vi "cell simulator - REAL TIME.vi"() -> ()   [LabVIEW 2017]
panel:
  in  "Tab Control":enum32{"SIMULATION"}(tab)
  in  "OK Button":bool
  in  "simulation setup":T1={"Setup test by"=2, "config value"=4.0, "time unit of panel"=0} {"time unit of panel" items=["seconds(s)", "minutes(min)", "hours(h)"]; "Setup test by" items=["Time(s)", "Current(A)", "C discharge"]}
  out "simulation conditions":T2
  out "time test":i32 format="%<%H:%M:%S>t"
  in  "Cell characteristics":T3={"temperature(ªC)\nbattery not used "=0.0, "N cycles"=0.0, "Time cell\nnot used(months)"=0.0, "Cycling temperature\nto K factors"=0, "capacity cell(Ah)"=10.0} {"Cycling temperature\nto K factors" items=["25ºC", "50ºC"]}
  out "Losses of capacity":T4
  in  "?":enum32{"PRINCIPAL GRAPH", "GRAPH DETAILS"}(tab)
  out "SOC(%)":dbl(slide) scale=0.0..100.0
  out "resolucion  \nSOC % / 1s":dbl
  out "principal graph":dynamicdata(graph)
  out "Vbat graph":dbl(graph)
  out "SOC graph":dbl(graph)
  out "C graph":dbl(graph)
  out "Current graph":dbl(graph)
  # "Vbat(V)"
  # "SOC(/)"
  # "C rate"
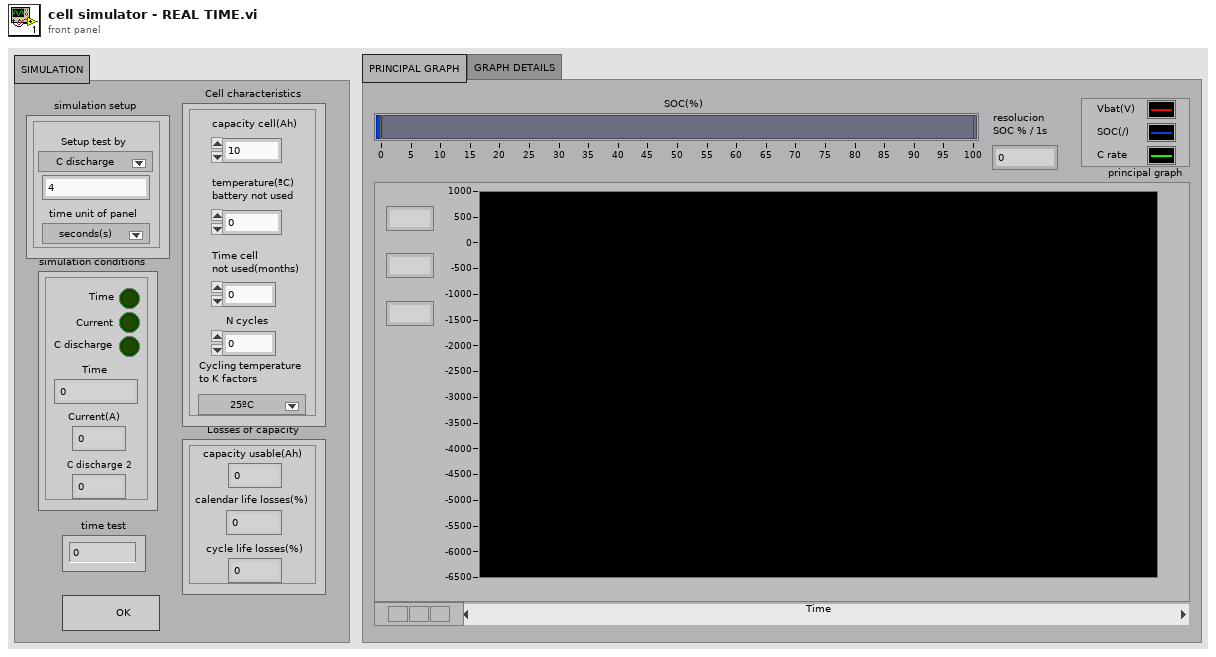
[diagram p1: front panel]
types:
  T1 = cluster{"Setup test by":u16, "config value":dbl, "time unit of panel":u16}
  T2 = cluster{"Time":bool, "Current":bool, "C discharge":bool, "Time":dbl, "Current(A)":dbl, "C discharge 2":dbl}
  T3 = cluster{"temperature(ªC)\nbattery not used ":dbl, "N cycles":dbl, "Time cell\nnot used(months)":dbl, "Cycling temperature\nto K factors":u16, "capacity cell(Ah)":dbl}
  T4 = cluster{"capacity usable(Ah)":dbl, "cycle life losses(%)":dbl, "calendar life losses(%)":dbl}
  T5 = cluster{" capacity usable(Ah)":dbl, " calendar life losses(%)":dbl, "cycle life losses(%)":dbl}
  T6 = cluster{"Time":bool, " Current":bool, "C discharge":bool, "Time(s)":dbl, "Current(A)":dbl, "C discharge":dbl}
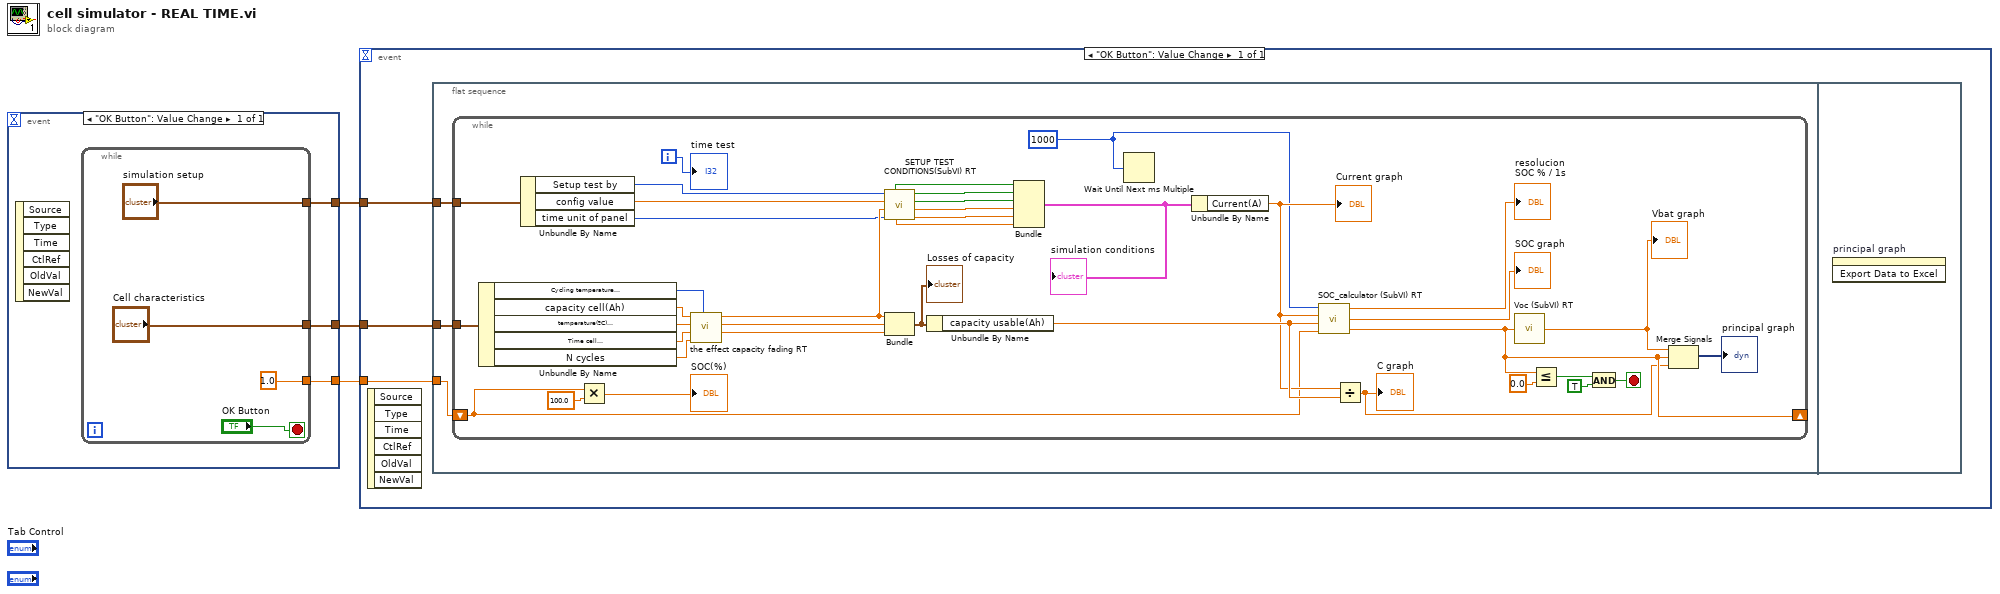
[diagram p0: block diagram]
diagram:
  n1 = event shown="[0] \"OK Button\": Value Change" {
    selector: _ -> [_]
    dyn-events: _ -> [_]
    timeout: _ -> [_]
    tunnel: [w6] -> w3
    tunnel: [w5] -> w2
    tunnel: [w4] -> w1
    event "OK Button": Value Change {
      n2 = event-data() -> ()  [unwired: 1 in, 6 out]
      n3 = while {
        tunnel: ["Cell characteristics"] -> w6
        tunnel: ["simulation setup"] -> w5
        tunnel: [1.0 ("Actual SOC( / )")] -> w4
        stop <- "OK Button" stop-if-true
      }
    }
  }
  n4 = event shown="[0] \"OK Button\": Value Change" {
    selector: _ -> [_]
    dyn-events: _ -> [_]
    timeout: _ -> [_]
    tunnel: w1 -> [w13]
    tunnel: w3 -> [w12]
    tunnel: w2 -> [w11]
    event "OK Button": Value Change {
      n5 = event-data() -> ()  [unwired: 1 in, 6 out]
      n6 = flat-sequence {
        tunnel: w13 -> [w16]
        tunnel: w12 -> [w15]
        tunnel: w11 -> [w14]
        frame #0 {
          n7 = while {
            shift-right: [w26] -> _
            shift-left: w16 -> [w24]
            tunnel: w15 -> [w30]
            tunnel: w14 -> [w29]
            i -> [w34]
            stop <- w27 stop-if-true
            w18 = u32 1000 ("millisecond multiple")
            n8 = Unbundle By Name(w30) -> ("Cycling temperature\nto K factors"=w52:u16, "capacity cell(Ah)"=w51:dbl, "temperature(ªC)\nbattery not used"=w50:dbl, "Time cell\nnot used(months)"=w49:dbl, "N cycles"=w48:dbl)
            n9 = Unbundle By Name(w29) -> ("Setup test by"=w47:u16, "config value"=w46:dbl, "time unit of panel"=w36:u16)
            n10 = Multiply(x=w24, y=100.0) -> (x*y=→"SOC(%)":dbl)
            n11 = call "the effect capacity fading RT.vi"("Cycling\ntemperature\nto K factors"=w52, "N cycles"=w48, "Time cell\nnot used(months)"=w49, "temperature(ªC) battery not used"=w50, "capacity cell"=w51) -> ("cycle life losses(%)"=w53:dbl, "calendar life losses(%)"=w54:dbl, "capacity usable(Ah)"=w45:dbl)  [unwired: 1 out]
            n12 = call "SETUP TEST CONDITIONS(SubVI) RT.vi"("setup time"=w36, "capacity usable(Ah)"=w45, "setup value"=w46, "setup test by"=w47) -> ("Current(A)"=w40:dbl, "Time(s)"=w41:dbl, 2:"C discharge"=w43:bool, "Current"=w44:bool, 4:"C discharge"=w39:dbl, "Time"=w42:bool)
            n13 = Bundle("capacity usable(Ah)"=w45, "calendar life losses(%)"=w54, "cycle life losses(%)"=w53) -> (w37:T5)  [unwired: 1 in]
            "Losses of capacity" <- w37
            n14 = Unbundle By Name(w37) -> ("capacity usable(Ah)"=w35:dbl)
            n15 = Bundle("Time"=w42, "Current"=w44, "C discharge"=w43, "Time(s)"=w41, "Current(A)"=w40, "C discharge"=w39) -> (w38:T6)  [unwired: 1 in]
            "simulation conditions" <- w38
            n16 = Wait Until Next ms Multiple(millisecond multiple=w18) -> ()  [unwired: 1 out]
            n17 = Unbundle By Name(w38) -> ("Current(A)"=w31:dbl)
            "Current graph" <- w31
            n18 = call "SOC_calculator (SubVI) RT.vi"("Pre SOC ( / )"=w24, "capacity usable(Ah)"=w35, "Current(A)"=w31, "tf integral (ms)"=w18) -> ("Actual SOC( / )"=w26:dbl, "SOC(%)"=→"SOC graph":dbl, "resolucion  \nSOC % / 1s"=→"resolucion  \nSOC % / 1s":dbl)
            n19 = Divide(x=w31, y=w35) -> (x/y=w17:dbl)
            "C graph" <- w17
            n20 = call "Voc (SubVI) RT.vi"("Actual SOC( / )"=w26) -> ("Voc"=w19:dbl)
            "Vbat graph" <- w19
            n21 = Less Or Equal?(x=w26, y=0.0) -> (x <= y?=w21:bool)
            n22 = And(x=w21, y=TRUE) -> (x .and. y?=w27:bool)
            n23 = Merge Signals(w19, w26, w17) -> (→"principal graph":dynamicdata)
            "time test" <- w34
          }
        }
        frame #1 {
          n24 = invoke on="principal graph" class="WFChart (strict)" method="Export Data to Excel"() -> ()  [unwired: 3 in, 3 out]
        }
      }
    }
  }
